vi "info.id & temp.vi"(7 "Espera acceso FT":u32, 8 "error out 2":errorcluster, 11 "ftHandle_out 2":u32) -> (0 "error out":errorcluster, 1 "ID":u64 format="%016x", 2 "Temperatura":dbl, 3 "ftHandle_out":u32)   [LabVIEW 2019]
panel:
  out "ID 2":u64 format="%0x"
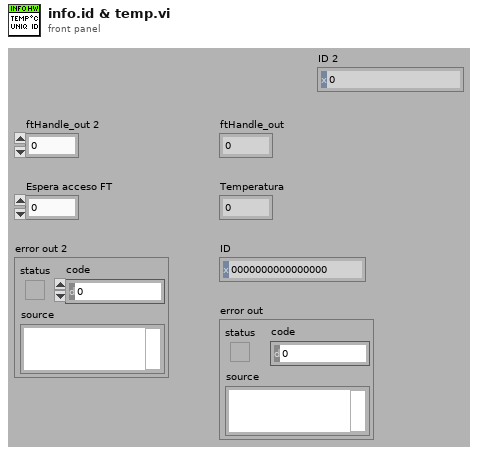
[diagram p1: front panel]
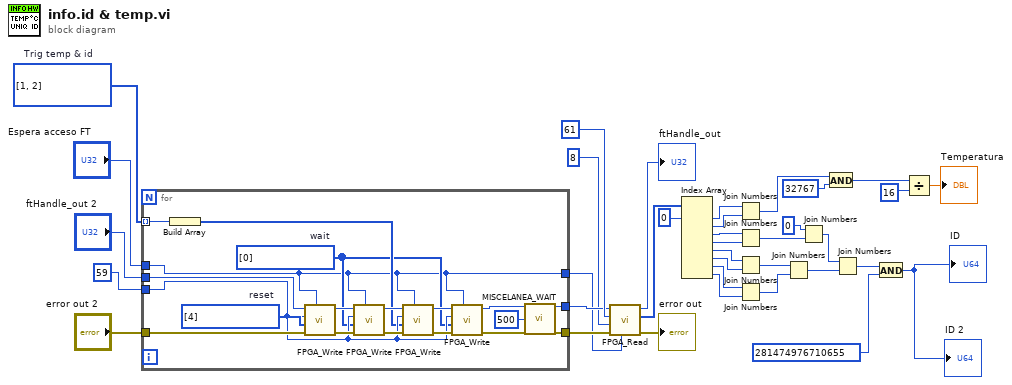
[diagram p0: block diagram]
diagram:
  w6 = u8[] [1, 2]  # Trig temp & id
  n1 = for {
    tunnel: w6 -> [w40] mode=indexing
    tunnel: u8 59 ("Dirección base") -> [w41]
    tunnel: "error out 2" -> [w54]
    tunnel: "ftHandle_out 2" -> [w53]
    tunnel: "Espera acceso FT" -> [w37]
    tunnel: [w46] -> w12
    tunnel: [w42] -> w11
    tunnel: [w37] -> w4
    w38 = i32[] [0]  # wait
    w52 = i32[] [4]  # reset
    n2 = Build Array(w40) -> (w39:u8[])
    n3 = call "FPGA_Write.vi"("Espera acceso USB"=w37, "error in"=w54, "Bytes de escritura"=w52, "Dirección base"=w41, "ftHandle_in"=w53) -> ("error out"=w50:errorcluster, "ftHandle_out"=w51:u32)  [unwired: 1 in, 2 out]
    n4 = call "FPGA_Write.vi"("Espera acceso USB"=w37, "error in"=w50, "Bytes de escritura"=w38, "Dirección base"=w41, "ftHandle_in"=w51) -> ("error out"=w49:errorcluster, "ftHandle_out"=w44:u32)  [unwired: 1 in, 2 out]
    n5 = call "FPGA_Write.vi"("Espera acceso USB"=w37, "error in"=w49, "Bytes de escritura"=w39, "Dirección base"=w41, "ftHandle_in"=w44) -> ("error out"=w48:errorcluster, "ftHandle_out"=w43:u32)  [unwired: 1 in, 2 out]
    n6 = call "FPGA_Write.vi"("Espera acceso USB"=w37, "error in"=w48, "Bytes de escritura"=w38, "Dirección base"=w41, "ftHandle_in"=w43) -> ("error out"=w47:errorcluster, "ftHandle_out"=w42:u32)  [unwired: 1 in, 2 out]
    n7 = call "MISCELANEA_WAIT.vi"("ms wait IN"=u32 500, "Error IN"=w47) -> ("Error OUT"=w46:errorcluster)  [unwired: 16 in, 1 out]
  }
  n8 = call "FPGA_Read.vi"("Espera acceso USB"=w4, "error in"=w12, "Numero Bytes"=u8 8, "Dirección base"=u8 61, "ftHandle_in"=w11) -> ("error out"=→"error out":errorcluster, "lpBuffer_out"=w14:u8[], "ftHandle_out"=→"ftHandle_out":u32)  [unwired: 2 in, 2 out]
  n9 = Index Array(array=w14, index #1=0 ("index")) -> (element #1=w16:u8, element #2=w17:u8, element #3=w29:u8, element #4=w30:u8, element #5=w31:u8, element #6=w32:u8, element #7=w33:u8, element #8=w34:u8)  [unwired: 7 in]
  n10 = Join Numbers(hi=w16, lo=w17) -> ((hi.lo)=w18:u16)
  n11 = Join Numbers(hi=w29, lo=w30) -> ((hi.lo)=w23:u16)
  n12 = Join Numbers(hi=w31, lo=w32) -> ((hi.lo)=w25:u16)
  n13 = Join Numbers(hi=w33, lo=w34) -> ((hi.lo)=w26:u16)
  n14 = Join Numbers(hi=w25, lo=w26) -> ((hi.lo)=w28:u32)
  n15 = Join Numbers(hi=u32 0, lo=w23) -> ((hi.lo)=w27:u64)
  n16 = And(x=w18, y=u16 32767) -> (x .and. y?=w20:u16)
  n17 = Join Numbers(hi=w27, lo=w28) -> ((hi.lo)=w3:u64)
  n18 = And(x=w3, y=u64 281474976710655) -> (x .and. y?=→"ID" →"ID 2":u64)
  n19 = Divide(x=w20, y=u16 16) -> (x/y=→"Temperatura":dbl)
